vi "Find index of the image name.vi"(8 "error in (no error)":errorcluster, 11 "Save Image in":refnum<class "Save Image.lvclass">) -> (0 "error out":errorcluster, 3 "Save Image out":refnum<class "Save Image.lvclass">)   [LabVIEW 2018, in "Save Image.lvclass"]
uses:
  Save Image.lvclass
  Simulated_Header/Simulated_Header.lvclass
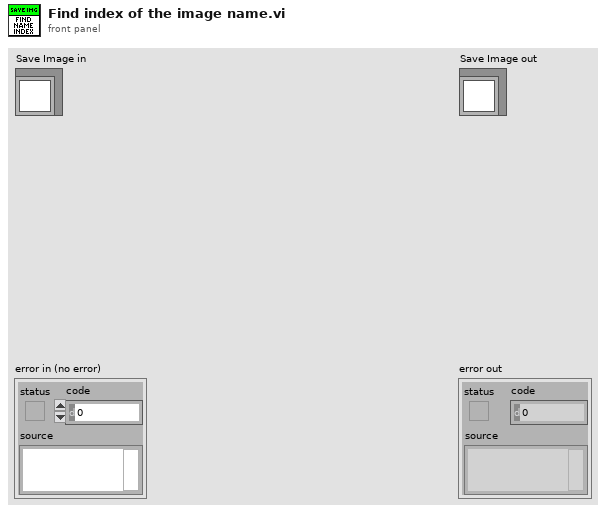
[diagram p1: front panel]
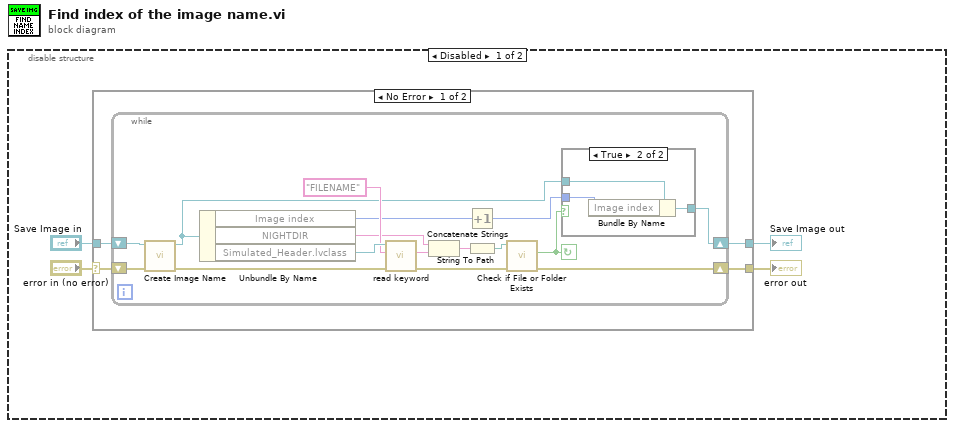
[diagram p0: block diagram]
diagram:
  n1 = disable-structure shown="Disabled" {
    frame Disabled {
      n2 = case shown="No Error" "error in (no error)" {
        selector: "error in (no error)" -> [w8 w30]
        tunnel: [w6 w30] -> w3
        tunnel: [w5 w29] -> w1
        tunnel: "Save Image in" -> [w7 w29]
        frame No Error {
          n3 = while {
            shift-right: [w11] -> w6
            shift-left: w8 -> [w24]
            shift-right: [w10] -> w5
            shift-left: w7 -> [w23]
            stop <- w9 continue-if-true
            n4 = call "Create Image Name.vi"("error in (no error)"=w24, "Save Image in"=w23) -> ("error out"=w21:errorcluster, "Save Image out"=w14:refnum<class "Save Image.lvclass">)  [unwired: 8 in]
            n5 = Unbundle By Name(w14) -> ("Image index"=w13:u32, "NIGHTDIR"=w18:string, "Simulated_Header.lvclass"=w22:refnum<class "Simulated_Header.lvclass">)
            n6 = call "read keyword.vi"("error in (no error)"=w21, "keyword"="FILENAME", "Simulated_Header in"=w22) -> ("error out"=w15:errorcluster, "value"=w19:string)  [unwired: 6 in, 1 out]
            n7 = Concatenate Strings(w18, w19) -> (w17:string)
            n8 = Increment(x=w13) -> (x+1=w12:u32)
            n9 = String To Path(string=w17) -> (path=w16:path)
            n10 = call <vilib>:"Check if File or Folder Exists.vi"("error in (no error)"=w15, "path"=w16) -> ("error out"=w11:errorcluster, "file or folder exists?"=w9:bool)  [unwired: 7 in, 1 out]
            n11 = case shown="True" w9 {
              tunnel: w14 -> [w25 w28]
              tunnel: w12 -> [_ w27]
              tunnel: [w25 w26] -> w10
              frame False {
              }
              frame True {
                n12 = Bundle By Name(cluster=w28, "Image index"=w27) -> (w26:refnum<class "Save Image.lvclass">)
              }
            }
          }
        }
        frame Error {
        }
      }
      "error out" <- w3
      "Save Image out" <- w1
    }
    frame Enabled {
    }
  }
